vi "Triggering Configuration.vi"(8 "error in (no error)":errorcluster, 11 "Node Ptr":T5 format="%.0x") -> (0 "error out":errorcluster)   [LabVIEW 2015, in "DMM-SWITCH-ScanList System Explorer.lvlib"]
uses:
  DMM-SWITCH-ScanList System Explorer.lvlib
  <vilib>/NI Veristand/Custom Device API/Custom Device Item Ref.ctl
  <instrlib>/niSwitch/niSwitch.LLB/niSwitch Trigger Input.ctl
  <instrlib>/niDMM/nidmm.llb/niDMM Measurement Complete.ctl
  <instrlib>/niDMM/nidmm.llb/niDMM Trigger.ctl
  <instrlib>/niSwitch/niSwitch.LLB/niSwitch Scan Advanced Output.ctl
  Shared/Constants.vi
  <vilib>/NI Veristand/Custom Device API/Get Item Property (U16).vi
  <vilib>/NI Veristand/Custom Device API/Set Item Property (U16).vi
  <vilib>/NI Veristand/Custom Device API/Custom Device API.lvlib
  Shared/DMM-SWITCH-ScanList Shared.lvlib
panel:
  in  "DMM Trigger Source":u16(ring)
  in  "DMM Measurement Complete":u16(ring)
  in  "Switch Scan Advanced Output":u16(ring)
  in  "Switch Trigger Source":u16(ring)
  in  "Switch Scan Advanced Output Type Def":T1=enum."TTL1" caption="Switch Scan Advanced Output"
  in  "DMM Trigger Source Type Def":T2=enum."TTL 1" caption="DMM Trigger Source"
  in  "DMM Measurement Complete Type Def":T3=enum."TTL 0" caption="DMM Measurement Complete"
  in  "SwitchTrigger Source Type Def":T4=enum."TTL0" caption="Switch Trigger Source"
  in  "Header":cluster{"Section Name":string}={"Section Name"="Custom Device Item Settings"}
  in  "Description":string
  in  "Name":string
  # "Triggers Configuration"
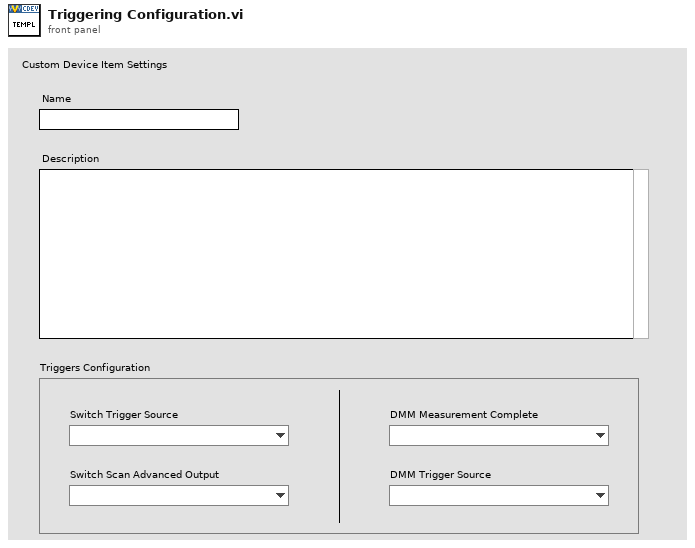
[diagram p1: front panel]
types:
  T1 = typedef "niSwitch Scan Advanced Output.ctl" = enum16{"None", "External", "TTL0", "TTL1", "TTL2", "TTL3", "TTL4", "TTL5", "TTL6", "TTL7", "ECL0", "ECL1", "PXI Star", "Rear Connector", "Front Connector", "Rear Connector Module 1", "Rear Connector Module 2", "Rear Connector Module 3", "Rear Connector Module 4", "Rear Connector Module 5", "Rear Connector Module 6", "Rear Connector Module 7", "Rear Connector Module 8", "Rear Connector Module 9", "Rear Connector Module 10", "Rear Connector Module 11", "Rear Connector Module 12", "Front Connector Module 1", "Front Connector Module 2", "Front Connector Module 3", "Front Connector Module 4", "Front Connector Module 5", "Front Connector Module 6", "Front Connector Module 7", "Front Connector Module 8", "Front Connector Module 9", "Front Connector Module 10", "Front Connector Module 11", "Front Connector Module 12"}
  T2 = typedef "niDMM Trigger.ctl" = enum16{"Immediate", "External", "TTL 0", "TTL 1", "TTL 2", "TTL 3", "TTL 4", "TTL 5", "TTL 6", "Software", "TTL 7", "PXI Star", "LBR Trig 1", "Aux Trig 1"}
  T3 = typedef "niDMM Measurement Complete.ctl" = enum16{"None", "External", "TTL 0", "TTL 1", "TTL 2", "TTL 3", "TTL 4", "TTL 5", "TTL 6", "TTL 7", "LBR Trig 0"}
  T4 = typedef "niSwitch Trigger Input.ctl" = enum16{"Immediate", "External", "TTL0", "TTL1", "TTL2", "TTL3", "TTL4", "TTL5", "TTL6", "TTL7", "ECL0", "ECL1", "PXI Star", "Software Trigger Function", "Rear Connector", "Front Connector", "Rear Connector of Module 1", "Rear Connector of Module 2", "Rear Connector of Module 3", "Rear Connector of Module 4", "Rear Connector of Module 5", "Rear Connector of Module 6", "Rear Connector of Module 7", "Rear Connector of Module 8", "Rear Connector of Module 9", "Rear Connector of Module 10", "Rear Connector of Module 11", "Rear Connector of Module 12", "Front Connector of Module 1", "Front Connector of Module 2", "Front Connector of Module 3", "Front Connector of Module 4", "Front Connector of Module 5", "Front Connector of Module 6", "Front Connector of Module 7", "Front Connector of Module 8", "Front Connector of Module 9", "Front Connector of Module 10", "Front Connector of Module 11", "Front Connector of Module 12"}
  T5 = typedef "Custom Device API.lvlib/Custom Device Item Ref.ctl" = u64
  T6 = typedef "Custom Device API.lvlib/Custom Device Item Info.ctl" = cluster{"Name":string, "Is Channel":bool, "GUID":string, "Is Waveform":bool}
  T7 = typedef "Custom Device API.lvlib/Custom Device Commands.ctl" = enum16{"Default", "Item renamed", "Shutdown", "Dynamic button pressed"}
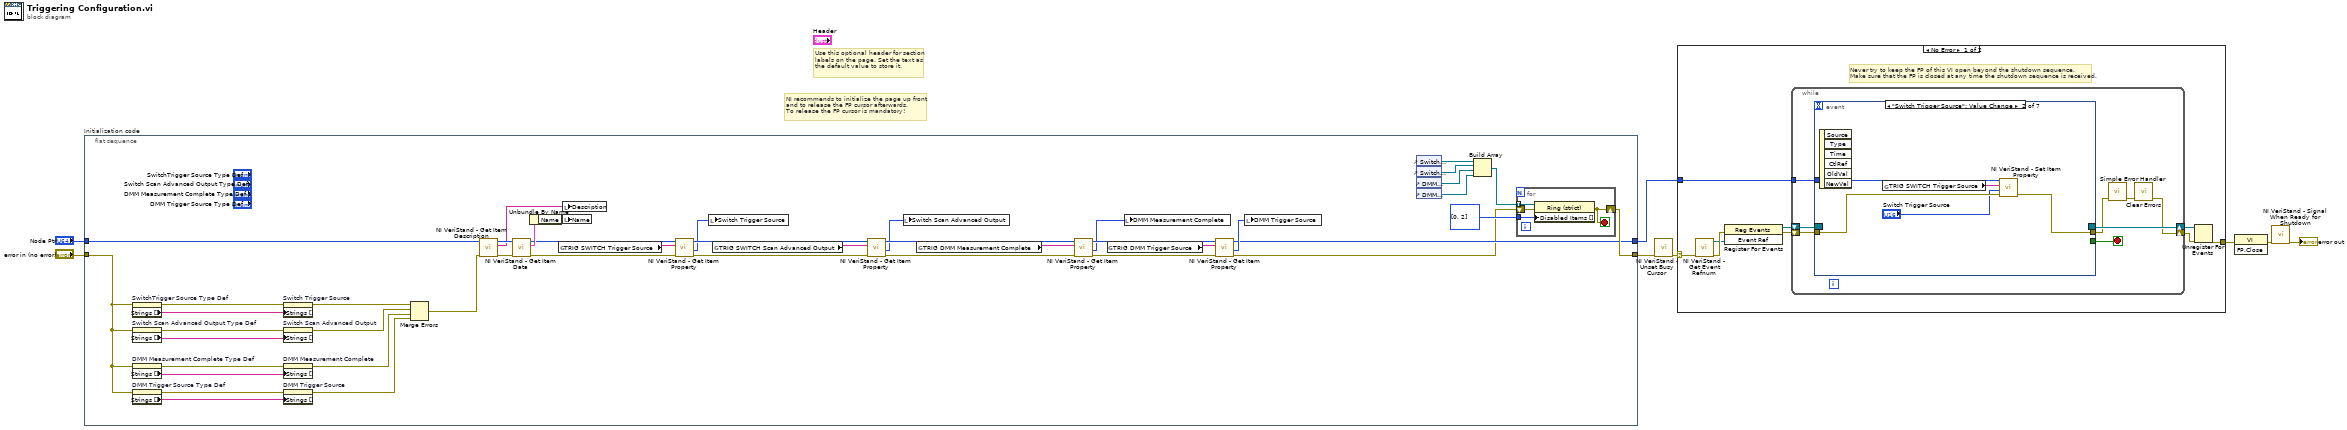
[diagram p0: block diagram]
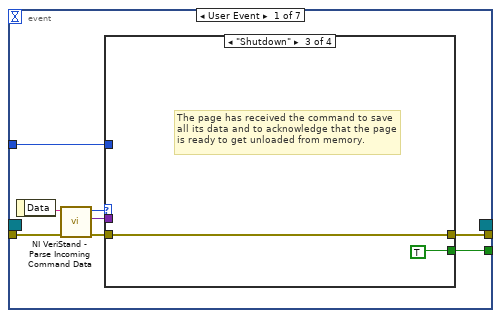
[diagram p2: hidden frame]
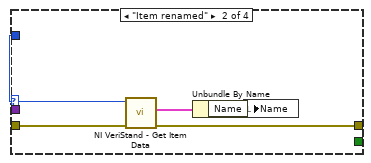
[diagram p4: hidden frame]
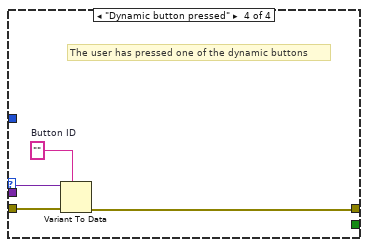
[diagram p5: hidden frame]
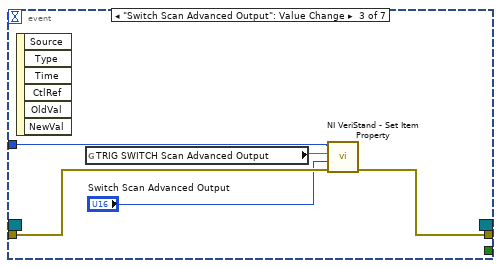
[diagram p6: hidden frame]
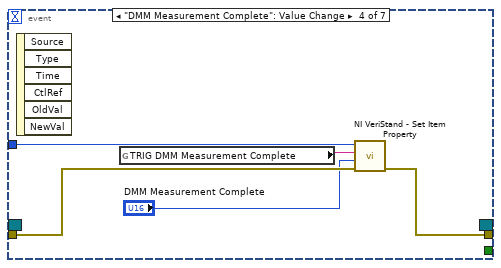
[diagram p7: hidden frame]
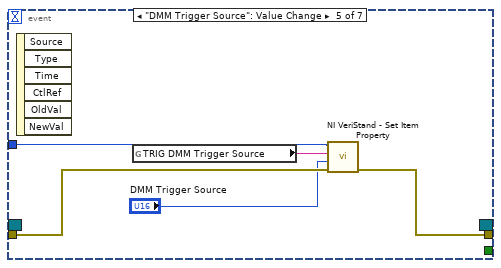
[diagram p8: hidden frame]
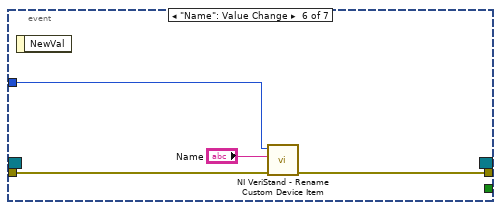
[diagram p9: hidden frame]
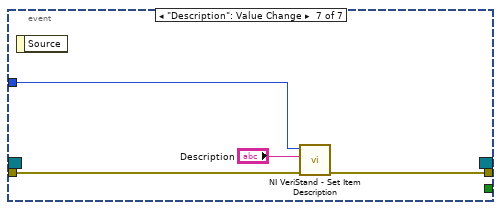
[diagram p10: hidden frame]
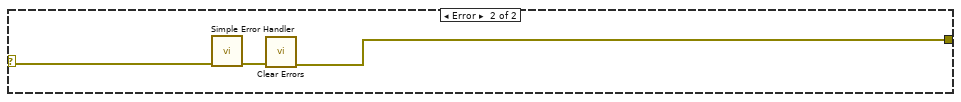
[diagram p11: hidden frame]
diagram:
  # "Use this optional header for section labels on the page. Set the text as the default value to store it."
  # "NI recommends to initialize the page up front\nand to release the FP cursor afterwards.\nTo release the FP cursor is mandatory!"
  n1 = flat-sequence "Initialization code" {
    tunnel: "error in (no error)" -> [w27]
    tunnel: "Node Ptr" -> [w52]
    tunnel: [w33] -> w4
    tunnel: [w28] -> w1
    frame #0 {
      n2 = property on="SwitchTrigger Source Type Def" class="Enum (strict)"(error in=w27) -> (error out=w19:errorcluster, "Strings []"=w25:string[])  [unwired: 1 in, 1 out]
      n3 = property on="Switch Scan Advanced Output Type Def" class="Enum (strict)"(error in=w27) -> (error out=w20:errorcluster, "Strings []"=w26:string[])  [unwired: 1 in, 1 out]
      n4 = property on="DMM Measurement Complete Type Def" class="Enum (strict)"(error in=w27) -> (error out=w21:errorcluster, "Strings []"=w24:string[])  [unwired: 1 in, 1 out]
      n5 = property on="DMM Trigger Source Type Def" class="Enum (strict)"(error in=w27) -> (error out=w22:errorcluster, "Strings []"=w23:string[])  [unwired: 1 in, 1 out]
      n6 = property on="Switch Trigger Source" class="Ring (strict)"(error in=w19, "Strings []"=w25) -> (error out=w18:errorcluster)  [unwired: 1 in, 1 out]
      n7 = property on="Switch Scan Advanced Output" class="Ring (strict)"(error in=w20, "Strings []"=w26) -> (error out=w17:errorcluster)  [unwired: 1 in, 1 out]
      n8 = property on="DMM Measurement Complete" class="Ring (strict)"(error in=w21, "Strings []"=w24) -> (error out=w16:errorcluster)  [unwired: 1 in, 1 out]
      n9 = property on="DMM Trigger Source" class="Ring (strict)"(error in=w22, "Strings []"=w23) -> (error out=w15:errorcluster)  [unwired: 1 in, 1 out]
      n10 = Merge Errors(w18, w17, w16, w15) -> (w10:errorcluster)
      n11 = call <vilib>:"NI VeriStand - Get Item Description.vi"("error in (no error)"=w10, "Item Ref in"=w52) -> ("error out"=w50:errorcluster, "Description"=w51:string, "Item Ref out"=w53:T5)  [unwired: 7 out]
      n12 = call <vilib>:"NI VeriStand - Get Item Data.vi"("error in (no error)"=w50, "Item Ref in"=w53) -> ("error out"=w41:errorcluster, "Item Info"=w49:T6, "Item Ref out"=w40:T5)  [unwired: 7 out]
      n13 = Unbundle By Name(w49) -> ("Name"=w48:string)
      n14 = global read "Constants.vi" "TRIG SWITCH Trigger Source"() -> (w32:string)
      n15 = local write "Description"(w51) -> ()
      n16 = local write "Name"(w48) -> ()
      n17 = call-poly <vilib>:"NI VeriStand - Get Item Property.vi"("error in (no error)"=w41, "Property Name"=w32, "Item Ref in"=w40) -> ("error out"=w45:errorcluster, "Value"=w39:u16, "Item Ref out"=w44:T5)  [unwired: 5 in, 1 out]
      n18 = local write "Switch Trigger Source"(w39) -> ()
      n19 = global read "Constants.vi" "TRIG SWITCH Scan Advanced Output"() -> (w31:string)
      n20 = call-poly <vilib>:"NI VeriStand - Get Item Property.vi"("error in (no error)"=w45, "Property Name"=w31, "Item Ref in"=w44) -> ("error out"=w47:errorcluster, "Value"=w36:u16, "Item Ref out"=w46:T5)  [unwired: 5 in, 1 out]
      n21 = local write "Switch Scan Advanced Output"(w36) -> ()
      n22 = global read "Constants.vi" "TRIG DMM Measurement Complete"() -> (w30:string)
      n23 = call-poly <vilib>:"NI VeriStand - Get Item Property.vi"("error in (no error)"=w47, "Property Name"=w30, "Item Ref in"=w46) -> ("error out"=w42:errorcluster, "Value"=w37:u16, "Item Ref out"=w43:T5)  [unwired: 5 in, 1 out]
      n24 = global read "Constants.vi" "TRIG DMM Trigger Source"() -> (w29:string)
      n25 = local write "DMM Measurement Complete"(w37) -> ()
      n26 = call-poly <vilib>:"NI VeriStand - Get Item Property.vi"("error in (no error)"=w42, "Property Name"=w29, "Item Ref in"=w43) -> ("error out"=w9:errorcluster, "Value"=w38:u16, "Item Ref out"=w28:T5)  [unwired: 5 in, 1 out]
      n27 = local write "DMM Trigger Source"(w38) -> ()
      n28 = control-ref of="Switch Trigger Source"() -> (w14:refnum<vi>)
      n29 = control-ref of="Switch Scan Advanced Output"() -> (w13:refnum<vi>)
      n30 = control-ref of="DMM Trigger Source"() -> (w12:refnum<vi>)
      n31 = control-ref of="DMM Measurement Complete"() -> (w11:refnum<vi>)
      n32 = Build Array(w14, w13, w12, w11) -> (w34:refnum<vi>[])
      n33 = for {
        tunnel: i32[] [0, 2] ("Disabled Items []") -> [w57]
        tunnel: w34 -> [w56] mode=indexing
        shift-right: [w54] -> w33
        shift-left: w9 -> [w55]
        stop <- w54 stop-if-true
        n34 = property class="Ring (strict)"(reference=w56, error in=w55, "Disabled Items []"=w57) -> (error out=w54:errorcluster)  [unwired: 1 out]
      }
    }
  }
  n35 = call <vilib>:"NI VeriStand - Unset Busy Cursor.vi"("error in (no error)"=w4) -> ("error out"=w3:errorcluster)  [unwired: 10 out]
  n36 = case shown="No Error" w3 {
    selector: w3 -> [w58 w125]
    tunnel: [w63 w123] -> w8
    tunnel: w1 -> [w59 _]
    frame No Error {
      # "Never try to keep the FP of this VI open beyond the shutdown sequence.\nMake sure that the FP is closed at any time the shutdown sequence is received."
      n37 = call <vilib>:"NI VeriStand - Get Event Refnum.vi"("error in (no error)"=w58) -> ("error out"=w66:errorcluster, "Event Ref"=w62:refnum<user-event>)  [unwired: 9 out]
      n38 = register-events(error in=w66, w62) -> (reference out=w60:refnum<event-registration>, error out=w61:errorcluster)  [unwired: 1 in]
      n39 = while {
        tunnel: w59 -> [w70]
        shift-right: [w67] -> w64
        shift-left: w61 -> [w73]
        shift-right: [w74] -> w65
        shift-left: w60 -> [w72]
        stop <- w71 stop-if-true
        n40 = event shown="[1] \"Switch Trigger Source\": Value Change" {
          selector: w72 -> [_ _ _ _ _ _ _]
          dyn-events: [_ _ _ _ _ _ _] -> w74
          timeout: _ -> [_ _ _ _ _ _ _]
          tunnel: w73 -> [w82 w98 w103 w108 w113 w118 w121]
          tunnel: [w78 _ _ _ _ _ _] -> w71
          tunnel: [w77 w97 w102 w107 w112 w117 w120] -> w69
          tunnel: w70 -> [w76 w99 w104 w109 w114 w116 w122]
          event User Event {
            n41 = event-data() -> ("Data"=w81:string)  [unwired: 1 out]
            n42 = call <vilib>:"NI VeriStand - Parse Incoming Command Data.vi"("error in (no error)"=w82, "Incoming data"=w81) -> ("error out"=w80:errorcluster, "Outgoing data"=w75:variant, "Action"=w79:T7)  [unwired: 7 out]
            n43 = case shown="\"Shutdown\"" w79 {
              tunnel: w80 -> [w83 w88 w89 w94]
              tunnel: [_ _ TRUE _] -> w78
              tunnel: [w83 w85 w89 w91] -> w77
              tunnel: w76 -> [_ w87 _ _]
              tunnel: w75 -> [_ _ _ w93]
              frame "Default", Default {
              }
              frame "Item renamed" {
                n44 = call <vilib>:"NI VeriStand - Get Item Data.vi"("error in (no error)"=w88, "Item Ref in"=w87) -> ("error out"=w85:errorcluster, "Item Info"=w86:T6)  [unwired: 8 out]
                n45 = Unbundle By Name(w86) -> ("Name"=w84:string)
                n46 = local write "Name"(w84) -> ()
              }
              frame "Shutdown" {
                # "The page has received the command to save all its data and to acknowledge that the page is ready to get unloaded from memory."
              }
              frame "Dynamic button pressed" {
                w92 = ""  # Button ID
                # "The user has pressed one of the dynamic buttons"
                n47 = Variant To Data(error in=w94, type=w92, Variant=w93) -> (error out=w91:errorcluster)  [unwired: 1 out]
              }
            }
          }
          event "Switch Trigger Source": Value Change {
            n48 = event-data() -> ()  [unwired: 7 out]
            n49 = global read "Constants.vi" "TRIG SWITCH Trigger Source"() -> (w96:string)
            n50 = call-poly <vilib>:"NI VeriStand - Set Item Property.vi"("error in (no error)"=w98, "Value"="Switch Trigger Source", "Property Name"=w96, "Item Ref in"=w99) -> ("error out"=w97:errorcluster)  [unwired: 5 in, 2 out]
          }
          event "Switch Scan Advanced Output": Value Change {
            n51 = event-data() -> ()  [unwired: 7 out]
            n52 = global read "Constants.vi" "TRIG SWITCH Scan Advanced Output"() -> (w101:string)
            n53 = call-poly <vilib>:"NI VeriStand - Set Item Property.vi"("error in (no error)"=w103, "Value"="Switch Scan Advanced Output", "Property Name"=w101, "Item Ref in"=w104) -> ("error out"=w102:errorcluster)  [unwired: 5 in, 2 out]
          }
          event "DMM Measurement Complete": Value Change {
            n54 = event-data() -> ()  [unwired: 7 out]
            n55 = global read "Constants.vi" "TRIG DMM Measurement Complete"() -> (w106:string)
            n56 = call-poly <vilib>:"NI VeriStand - Set Item Property.vi"("error in (no error)"=w108, "Value"="DMM Measurement Complete", "Property Name"=w106, "Item Ref in"=w109) -> ("error out"=w107:errorcluster)  [unwired: 5 in, 2 out]
          }
          event "DMM Trigger Source": Value Change {
            n57 = event-data() -> ()  [unwired: 7 out]
            n58 = global read "Constants.vi" "TRIG DMM Trigger Source"() -> (w111:string)
            n59 = call-poly <vilib>:"NI VeriStand - Set Item Property.vi"("error in (no error)"=w113, "Value"="DMM Trigger Source", "Property Name"=w111, "Item Ref in"=w114) -> ("error out"=w112:errorcluster)  [unwired: 5 in, 2 out]
          }
          event "Name": Value Change {
            n60 = event-data() -> ()  [unwired: 2 out]
            n61 = call <vilib>:"NI VeriStand - Rename Custom Device Item.vi"("error in (no error)"=w118, "New Name"="Name", "Item Ref in"=w116) -> ("error out"=w117:errorcluster)  [unwired: 1 in, 7 out]
          }
          event "Description": Value Change {
            n62 = event-data() -> ()  [unwired: 2 out]
            n63 = call <vilib>:"NI VeriStand - Set Item Description.vi"("error in (no error)"=w121, "Description"="Description", "Item Ref in"=w122) -> ("error out"=w120:errorcluster)  [unwired: 8 out]
          }
        }
        n64 = call <vilib>:"Simple Error Handler.vi"("error in (no error)"=w69) -> ("error out"=w68:errorcluster)  [unwired: 1 in, 7 out]
        n65 = call <vilib>:"Clear Errors.vi"("error in (no error)"=w68) -> ("error out"=w67:errorcluster)  [unwired: 1 in, 5 out]
      }
      n66 = Unregister For Events(event registration refnum=w65, error in=w64) -> (error out=w63:errorcluster)
    }
    frame Error {
      n67 = call <vilib>:"Simple Error Handler.vi"("error in (no error)"=w125) -> ("error out"=w124:errorcluster)  [unwired: 1 in, 7 out]
      n68 = call <vilib>:"Clear Errors.vi"("error in (no error)"=w124) -> ("error out"=w123:errorcluster)  [unwired: 1 in, 5 out]
    }
  }
  n69 = invoke class="VI" method="FP.Close"(error in=w8) -> (error out=w7:errorcluster)  [unwired: 2 in, 2 out]
  n70 = call <vilib>:"NI VeriStand - Signal When Ready for Shutdown.vi"("error in (no error)"=w7) -> ("error out"=→"error out":errorcluster)  [unwired: 10 out]
